vi "FPGA_DIOReadSlowValueRelayRev.vi"(8 "error in (no error)":errorcluster, 11 "DIODeviceRef In":T1) -> (0 "error out":errorcluster, 2 "Relay Reverse":u8, 3 "DIODeviceRef Out":T1)   [LabVIEW 2017]
uses:
  <vilib>/Rock Robotics/SystemInterfaces/DIO/FPGA_DIODevRef.ctl
  <vilib>/Rock Robotics/SystemInterfaces/System/FPGA_SystemFPGA Ref Global.vi
  <vilib>/Utility/error.llb/Error Cluster From Error Code.vi
  <vilib>/rvi/errors/niLvFpgaAdjustHostInterfaceError.vi
  <vilib>/rvi/interface/nirviReadWriteControl/nirviReadWriteControl.xnode
  <vilib>/Rock Robotics/SystemInterfaces/System/FPGA_SystemFRC FPGA Ref.ctl
  NiFpgaLv.dll
  <vilib>/rvi/interface/Simulation/niFpgaSimulationCallBeginRW.vi
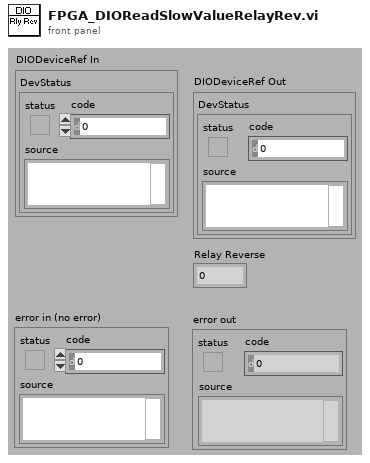
[diagram p1: front panel]
types:
  T1 = typedef "FPGA_DIODevRef.ctl" = cluster{"DevStatus":errorcluster}
  T2 = typedef "FPGA_SystemFRC FPGA Ref.ctl" = refnum<k20>
  T3 = cluster{"Forward":fxp<+,4,4>, "Reverse":fxp<+,4,4>}
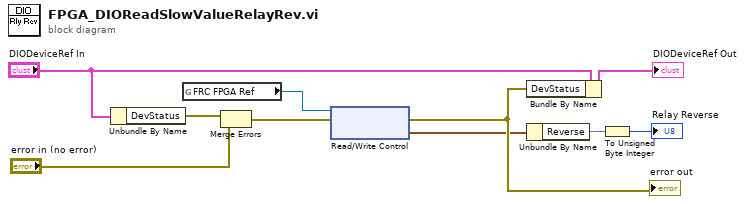
[diagram p0: block diagram]
diagram:
  n1 = Unbundle By Name("DIODeviceRef In") -> ("DevStatus"=w5:errorcluster)
  n2 = global read "FPGA_SystemFPGA Ref Global.vi" "FRC FPGA Ref"() -> (w3:T2)
  n3 = Merge Errors(w5, "error in (no error)") -> (w4:errorcluster)
  n4 = xnode "Read/Write Control"("FPGA VI Reference In"=w3, "error in"=w4) -> ("error out"=w8:errorcluster, "Relay.Value"=w6:T3)  [unwired: 1 out]
  "error out" <- w8
  n5 = Bundle By Name(cluster="DIODeviceRef In", "DevStatus"=w8) -> (→"DIODeviceRef Out":T1)
  n6 = Unbundle By Name(w6) -> ("Reverse"=w7:fxp<+,4,4>)
  n7 = To Unsigned Byte Integer(number=w7) -> (unsigned 8bit integer=→"Relay Reverse":u8)
